vi "checkforground.vi"(1 "Vertical coupling":i32) -> (0 "If GND; set in AC mode (GND mode will be fixed later)":i32)   [LabVIEW 2011]
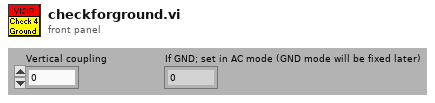
[diagram p1: front panel]
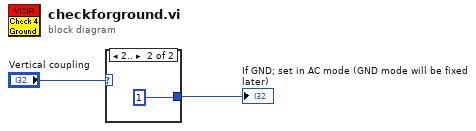
[diagram p0: block diagram]
diagram:
  n1 = case shown="2.." "Vertical coupling" {
    selector: "Vertical coupling" -> [w3 _]
    tunnel: [w3 1 ("Vertical coupling")] -> w1
    frame ..1, Default {
    }
    frame 2.. {
    }
  }
  "If GND; set in AC mode (GND mode will be fixed later)" <- w1
